vi "INTELLIFAUCET Driver.vi"(0 "Test Fixture Hardware":T2={"Power "={"Yokogawa"={"WT210"={"Sample Rate (1: 0.25s)"=1, "A Range (12: 20A)"=11, "V Range (6: 600V)"=4, "Power VISA Yokogawa WT210"="WT210"}, "WT500"={"Power VISA Yokogawa WT500"="", "V Range (8: 1000V)"=6, "I Range (7: 40A)"=7, "Update Rate (3: 500ms)"=2}, "WT310_2"={"Sample Rate (1: 0.25s)"=1, "A Range (12: 20A)"=11, "V Range (6: 600V)"=4, "Power VISA Yokogawa WT310_2"="WT310_2"}, "WT310_3"={"Sample Rate (1: 0.25s)"=1, "A Range (12: 20A)"=11, "V Range (6: 600V)"=4, "Power VISA Yokogawa WT310_3"="WT310_3"}}, "Aplus"={"Aplus IP Address"="192.168.1.101", "Remote Port"=502, "Instrument"="APLUS", "Instr Driver Revision"="1.03.0053"}, "Power Limits"={"Crest Factor"={"Upper Limit"=1.49, "Lower Limit"=1.34}, "Harmonic Content"={"Uthd"=2.0}, "Voltage"={"% Error"=2.0}, "Stability"={"<1 Watt "={"Wattage"=1.0, "Slope (mW/H)"=10.0}, ">1 Watt"={"1%Power/Hour"=1.0}}}, "Nominal Voltage"=120, "Time Limit (s)"=10800.0, "Power Variation Limit (%)"=50.0, "Power Supply"={"Chroma 61605"="CHROMA", "Use Chroma?"=FALSE}}, "Weight Scale"={"Com Options"={"IND560Scale VISA"="IND560", "IP Address"="", "Remote Port"=502, "Setra Scale VISA"="SETRA", "GSE 350"="GSE350"}, "Select Scale"=""}, "Flow Rates"={"Laurel Cold IP Address"="", "Laurel Hot IP Address"="", "Hot Water Laurel VISA"="LaurelMeter_Hot", "Cold Water Laurel VISA"="LaurelMeter_Cold", "Remote Port"=0, "Laurel Communication Type"="", "Meters To Collect (Hot Cold)"="", "HOT Laurel Reference"=refnum, "COLD Laurel Reference"=refnum}, "Analog Data"={"Agilent"={"Agilent 34972_1"="34972A_1", "Agilent 34972_2"="34972A_2", "Agilent 34972_3"="34972A_3", "Agilent 34972_4"="34972A_3", "Agilent 34972_5"="34972A_3", "Agilent 34972_6"="34972A_3", "Agilent Gain"=0.0, "TC Type (K,J,T)"="", "Instrument IDN?"="", "TC Channels-List"="", "Analog Channels-List"="", "Agilent Cluster Array"=[], "TC Channels-List 2"="", "Analog Channels-List 2"=""}, "Yokogawa"={"MW100"="MW100", "Intellifaucet"=FALSE}, "Select Analog"="", "TC Coefficients"={"TC Coefficients 1"=[], "TC Coefficients 2"=[], "TC Coefficients 3"=[], "TC Coefficients 4"=[], "TC Coefficients 5"=[], "TC Coefficients 6"=[], "TC Coefficients 7"=[]}, "NI Tasks (Dryer DOE)"=["TC Temps-Module 1", "TC Temps-Module 2", "TC Temps-Module 3", "TC Temps-Module 4", "TC Temps-Module 5", "Gas and Temp-Module 6", "AC_DC Events-Module 7"], "Laurel Analog"={"Laurel IP (Water Temp)"="", "Laurel IP (Pressure)"=""}}, "ITHX-Temp Humidity"={"IP Address 1"="", "Remote Port"=0, "IP Address 2"="", "IP Address 3"=""}, "Gas Meter"={"Gas Meter 1"="GasMeter1", "Gas Meter 2"="COM4", "Gas Meter 3"="COM5", "Gas Meter 4"="COM6", "Gas Meter 5"="COM7", "Gas Meter 6"="COM8", "Data Frame Format"={"Absolute Pressure"=FALSE, "Gauge/Diff. Pressure"=FALSE, "Barometric Pressure"=FALSE, "Temperature"=FALSE, "Volumetric"=FALSE, "Mass"=FALSE, "Setpoint"=FALSE, "Valve Drive"=FALSE, "Totalizer"=FALSE, "Totalizer Timer"=FALSE, "Totalizer Average Flow"=FALSE, "Totalizer Peak Flow"=FALSE, "Gas Selected"=FALSE, "Tot. Timer Format"=0}, "Measurement Data"={"Absolute Pressure"=0.0, "Gauge/Diff. Pressure"=0.0, "Barometric Pressure"=0.0, "Temperature"=0.0, "Volumetric Flow"=0.0, "Mass Flow"=0.0, "Setpoint"=0.0, "Valve Drive"=0.0, "Totalizer"=0.0, "[hr]"=0.0, "[min]"=0.0, "[sec]"=0.0, "Totalizer Average Flow"=0.0, "Totalizer Peak Flow"=0.0, "Gas selected"=""}, "Measurement Units"={"Software Rev"="", "Model Number"="", "Manufacturer Info"="", "Software Sub-Rev"="", "Board Rev"="", "Units of Measure Input"={"Abs. Pressure"="", "Gauge/Diff. Press."="", "Barometric Press."="", "Temperature"="", "Volume"="", "Mass"="", "Setpoint"="", "Valve Drive"="", "Totalizer"="", "Tot. Timer"="", "Tot. Avg. Flow"="", "Tot. Peak Flow"=""}}}, "Barometric Pressure"={"HEISE 901A"="HEISE", "Use Barometer?"=FALSE}, "Gas Analysis"={"Ultramat 23 VISA"="ULTRAMAT"}, "Inficon Micro GC"={"Propane IP Address"="192.168.1.33", "Natural Gas  IP Address"="192.168.1.32", "Remote Port"=502}} {"Power"."Yokogawa"."WT310_3"."V Range (6: 600V)" items=["Auto", "15V", "30V", "60V", "150V", "300V", "600V"]; "Power"."Yokogawa"."WT310_3"."A Range (12: 20A)" items=["Auto", "5mA", "10mA", "20mA", "50mA", "100mA", "200mA", "0.5A", "1A", "2A", "5A", "10A", "20A", "50mV", "100mV", "200mV", "2.5V", "5V", "10V"]; "Power"."Yokogawa"."WT310_3"."Sample Rate (1: 0.25s)" items=["0.1s", "0.25s", "0.5s", "1s", "2s", "5s"]; "Power"."Yokogawa"."WT310_2"."V Range (6: 600V)" items=["Auto", "15V", "30V", "60V", "150V", "300V", "600V"]; "Power"."Yokogawa"."WT310_2"."A Range (12: 20A)" items=["Auto", "5mA", "10mA", "20mA", "50mA", "100mA", "200mA", "0.5A", "1A", "2A", "5A", "10A", "20A", "50mV", "100mV", "200mV", "2.5V", "5V", "10V"]; "Power"."Yokogawa"."WT310_2"."Sample Rate (1: 0.25s)" items=["0.1s", "0.25s", "0.5s", "1s", "2s", "5s"]; "Power"."Yokogawa"."WT500"."Update Rate (3: 500ms)" items=["-", "100ms", "200ms", "500ms", "1s", "2s", "5s"]; "Power"."Yokogawa"."WT500"."I Range (7: 40A)" items=["AUTO", "500 mA", "1 A", "2 A", "5 A", "10 A", "20 A", "40 A", "S-AUTO", "50 mV", "100 mV", "200 mV", "500 mV", "1 V", "2 V", "5 V", "10 V", "250 mA", "500 mA", "1 A", "2.5 A", "5 A", "10 A", "20 A", "25 mV", "50 mV", "100 mV", "250 mV", "500 mV", "1 V", "2.5 V", "5 V"]; "Power"."Yokogawa"."WT500"."V Range (8: 1000V)" items=["AUTO", "15", "30", "60", "100", "150", "300", "600", "1000", "7.5", "15", "30", "50", "75", "150", "300", "500"]; "Power"."Yokogawa"."WT210"."V Range (6: 600V)" items=["Auto", "15V", "30V", "60V", "150V", "300V", "600V"]; "Power"."Yokogawa"."WT210"."A Range (12: 20A)" items=["Auto", "5mA", "10mA", "20mA", "50mA", "100mA", "200mA", "0.5A", "1A", "2A", "5A", "10A", "20A", "50mV", "100mV", "200mV", "2.5V", "5V", "10V"]; "Power"."Yokogawa"."WT210"."Sample Rate (1: 0.25s)" items=["0.1s", "0.25s", "0.5s", "1s", "2s", "5s"]}, 1 "Mode":T13=enum."Stop Flow", 2 "Use General Conversion":bool, 3 "TEMP,FLOW":T1, 5 "Temperature(F)":dbl(slide)=58.0 scale=40.0..120.0, 7 "Flow Rate (GPM)":dbl(slide)=100.0 scale=0.0..100.0, 9 "uA Set":i32, 11 "Error In":errorcluster, 12 "Debug":bool, 13 "Refnum in":T12, 14 "Use Proportion Valve":bool) -> (4 "Test Fixture Hardware Output":T2={"Power "={"Yokogawa"={"WT210"={"Sample Rate (1: 0.25s)"=1, "A Range (12: 20A)"=11, "V Range (6: 600V)"=4, "Power VISA Yokogawa WT210"="WT210"}, "WT500"={"Power VISA Yokogawa WT500"="", "V Range (8: 1000V)"=6, "I Range (7: 40A)"=7, "Update Rate (3: 500ms)"=2}, "WT310_2"={"Sample Rate (1: 0.25s)"=1, "A Range (12: 20A)"=11, "V Range (6: 600V)"=4, "Power VISA Yokogawa WT310_2"="WT310_2"}, "WT310_3"={"Sample Rate (1: 0.25s)"=1, "A Range (12: 20A)"=11, "V Range (6: 600V)"=4, "Power VISA Yokogawa WT310_3"="WT310_3"}}, "Aplus"={"Aplus IP Address"="192.168.1.101", "Remote Port"=502, "Instrument"="APLUS", "Instr Driver Revision"="1.03.0053"}, "Power Limits"={"Crest Factor"={"Upper Limit"=1.49, "Lower Limit"=1.34}, "Harmonic Content"={"Uthd"=2.0}, "Voltage"={"% Error"=2.0}, "Stability"={"<1 Watt "={"Wattage"=1.0, "Slope (mW/H)"=10.0}, ">1 Watt"={"1%Power/Hour"=1.0}}}, "Nominal Voltage"=120, "Time Limit (s)"=10800.0, "Power Variation Limit (%)"=50.0, "Power Supply"={"Chroma 61605"="CHROMA", "Use Chroma?"=FALSE}}, "Weight Scale"={"Com Options"={"IND560Scale VISA"="IND560", "IP Address"="", "Remote Port"=502, "Setra Scale VISA"="SETRA", "GSE 350"="GSE350"}, "Select Scale"=""}, "Flow Rates"={"Laurel Cold IP Address"="", "Laurel Hot IP Address"="", "Hot Water Laurel VISA"="LaurelMeter_Hot", "Cold Water Laurel VISA"="LaurelMeter_Cold", "Remote Port"=0, "Laurel Communication Type"="", "Meters To Collect (Hot Cold)"="", "HOT Laurel Reference"=refnum, "COLD Laurel Reference"=refnum}, "Analog Data"={"Agilent"={"Agilent 34972_1"="34972A_1", "Agilent 34972_2"="34972A_2", "Agilent 34972_3"="34972A_3", "Agilent 34972_4"="34972A_3", "Agilent 34972_5"="34972A_3", "Agilent 34972_6"="34972A_3", "Agilent Gain"=0.0, "TC Type (K,J,T)"="", "Instrument IDN?"="", "TC Channels-List"="", "Analog Channels-List"="", "Agilent Cluster Array"=[], "TC Channels-List 2"="", "Analog Channels-List 2"=""}, "Yokogawa"={"MW100"="MW100", "Intellifaucet"=FALSE}, "Select Analog"="", "TC Coefficients"={"TC Coefficients 1"=[], "TC Coefficients 2"=[], "TC Coefficients 3"=[], "TC Coefficients 4"=[], "TC Coefficients 5"=[], "TC Coefficients 6"=[], "TC Coefficients 7"=[]}, "NI Tasks (Dryer DOE)"=["TC Temps-Module 1", "TC Temps-Module 2", "TC Temps-Module 3", "TC Temps-Module 4", "TC Temps-Module 5", "Gas and Temp-Module 6", "AC_DC Events-Module 7"], "Laurel Analog"={"Laurel IP (Water Temp)"="", "Laurel IP (Pressure)"=""}}, "ITHX-Temp Humidity"={"IP Address 1"="", "Remote Port"=0, "IP Address 2"="", "IP Address 3"=""}, "Gas Meter"={"Gas Meter 1"="GasMeter1", "Gas Meter 2"="COM4", "Gas Meter 3"="COM5", "Gas Meter 4"="COM6", "Gas Meter 5"="COM7", "Gas Meter 6"="COM8", "Data Frame Format"={"Absolute Pressure"=FALSE, "Gauge/Diff. Pressure"=FALSE, "Barometric Pressure"=FALSE, "Temperature"=FALSE, "Volumetric"=FALSE, "Mass"=FALSE, "Setpoint"=FALSE, "Valve Drive"=FALSE, "Totalizer"=FALSE, "Totalizer Timer"=FALSE, "Totalizer Average Flow"=FALSE, "Totalizer Peak Flow"=FALSE, "Gas Selected"=FALSE, "Tot. Timer Format"=0}, "Measurement Data"={"Absolute Pressure"=0.0, "Gauge/Diff. Pressure"=0.0, "Barometric Pressure"=0.0, "Temperature"=0.0, "Volumetric Flow"=0.0, "Mass Flow"=0.0, "Setpoint"=0.0, "Valve Drive"=0.0, "Totalizer"=0.0, "[hr]"=0.0, "[min]"=0.0, "[sec]"=0.0, "Totalizer Average Flow"=0.0, "Totalizer Peak Flow"=0.0, "Gas selected"=""}, "Measurement Units"={"Software Rev"="", "Model Number"="", "Manufacturer Info"="", "Software Sub-Rev"="", "Board Rev"="", "Units of Measure Input"={"Abs. Pressure"="", "Gauge/Diff. Press."="", "Barometric Press."="", "Temperature"="", "Volume"="", "Mass"="", "Setpoint"="", "Valve Drive"="", "Totalizer"="", "Tot. Timer"="", "Tot. Avg. Flow"="", "Tot. Peak Flow"=""}}}, "Barometric Pressure"={"HEISE 901A"="HEISE", "Use Barometer?"=FALSE}, "Gas Analysis"={"Ultramat 23 VISA"="ULTRAMAT"}, "Inficon Micro GC"={"Propane IP Address"="192.168.1.33", "Natural Gas  IP Address"="192.168.1.32", "Remote Port"=502}} {"Power"."Yokogawa"."WT310_3"."V Range (6: 600V)" items=["Auto", "15V", "30V", "60V", "150V", "300V", "600V"]; "Power"."Yokogawa"."WT310_3"."A Range (12: 20A)" items=["Auto", "5mA", "10mA", "20mA", "50mA", "100mA", "200mA", "0.5A", "1A", "2A", "5A", "10A", "20A", "50mV", "100mV", "200mV", "2.5V", "5V", "10V"]; "Power"."Yokogawa"."WT310_3"."Sample Rate (1: 0.25s)" items=["0.1s", "0.25s", "0.5s", "1s", "2s", "5s"]; "Power"."Yokogawa"."WT310_2"."V Range (6: 600V)" items=["Auto", "15V", "30V", "60V", "150V", "300V", "600V"]; "Power"."Yokogawa"."WT310_2"."A Range (12: 20A)" items=["Auto", "5mA", "10mA", "20mA", "50mA", "100mA", "200mA", "0.5A", "1A", "2A", "5A", "10A", "20A", "50mV", "100mV", "200mV", "2.5V", "5V", "10V"]; "Power"."Yokogawa"."WT310_2"."Sample Rate (1: 0.25s)" items=["0.1s", "0.25s", "0.5s", "1s", "2s", "5s"]; "Power"."Yokogawa"."WT500"."Update Rate (3: 500ms)" items=["-", "100ms", "200ms", "500ms", "1s", "2s", "5s"]; "Power"."Yokogawa"."WT500"."I Range (7: 40A)" items=["AUTO", "500 mA", "1 A", "2 A", "5 A", "10 A", "20 A", "40 A", "S-AUTO", "50 mV", "100 mV", "200 mV", "500 mV", "1 V", "2 V", "5 V", "10 V", "250 mA", "500 mA", "1 A", "2.5 A", "5 A", "10 A", "20 A", "25 mV", "50 mV", "100 mV", "250 mV", "500 mV", "1 V", "2.5 V", "5 V"]; "Power"."Yokogawa"."WT500"."V Range (8: 1000V)" items=["AUTO", "15", "30", "60", "100", "150", "300", "600", "1000", "7.5", "15", "30", "50", "75", "150", "300", "500"]; "Power"."Yokogawa"."WT210"."V Range (6: 600V)" items=["Auto", "15V", "30V", "60V", "150V", "300V", "600V"]; "Power"."Yokogawa"."WT210"."A Range (12: 20A)" items=["Auto", "5mA", "10mA", "20mA", "50mA", "100mA", "200mA", "0.5A", "1A", "2A", "5A", "10A", "20A", "50mV", "100mV", "200mV", "2.5V", "5V", "10V"]; "Power"."Yokogawa"."WT210"."Sample Rate (1: 0.25s)" items=["0.1s", "0.25s", "0.5s", "1s", "2s", "5s"]}, 8 "uA Output":i32, 15 "Error Out":errorcluster)   [LabVIEW 2019]
uses:
  Type Definitions/INTELLIFAUCET Set Mode.ctl
  Washer DOE/Type Definitions/DOE Test Fixture Hardware.ctl
  Utility/Type Definitions/UTILITY Power Inputs Control.ctl
  Drivers/IND560 Scale Monitor/Type Definitions/IND560 Configuration.ctl
  Type Definitions/HEWH Agilent Cluster.ctl
  Utility/Type Definitions/UTILITY TC Coefficients.ctl
  Drivers/Omega FMA-1600A Series Gas Flow Meter/Type Definitions/FMA1600A COM Ports.ctl
  Drivers/Alicat Gas Meter Driver/Sub-VIs/Data Frame.ctl
  Drivers/Alicat Gas Meter Driver/Sub-VIs/Data Cluster.ctl
  Drivers/Omega FMA-1600A Series Gas Flow Meter/Type Definitions/FMA1600A Units String.ctl
  Drivers/Alicat Gas Meter Driver/Sub-VIs/Units of Measure.ctl
  Type Definitions/INTELLIFAUCT Temp Flow.ctl
panel:
  in  "milliseconds to wait":u32=75
  # "%"
  # "Totalizer Timer"
  # "Totalizer Timer"
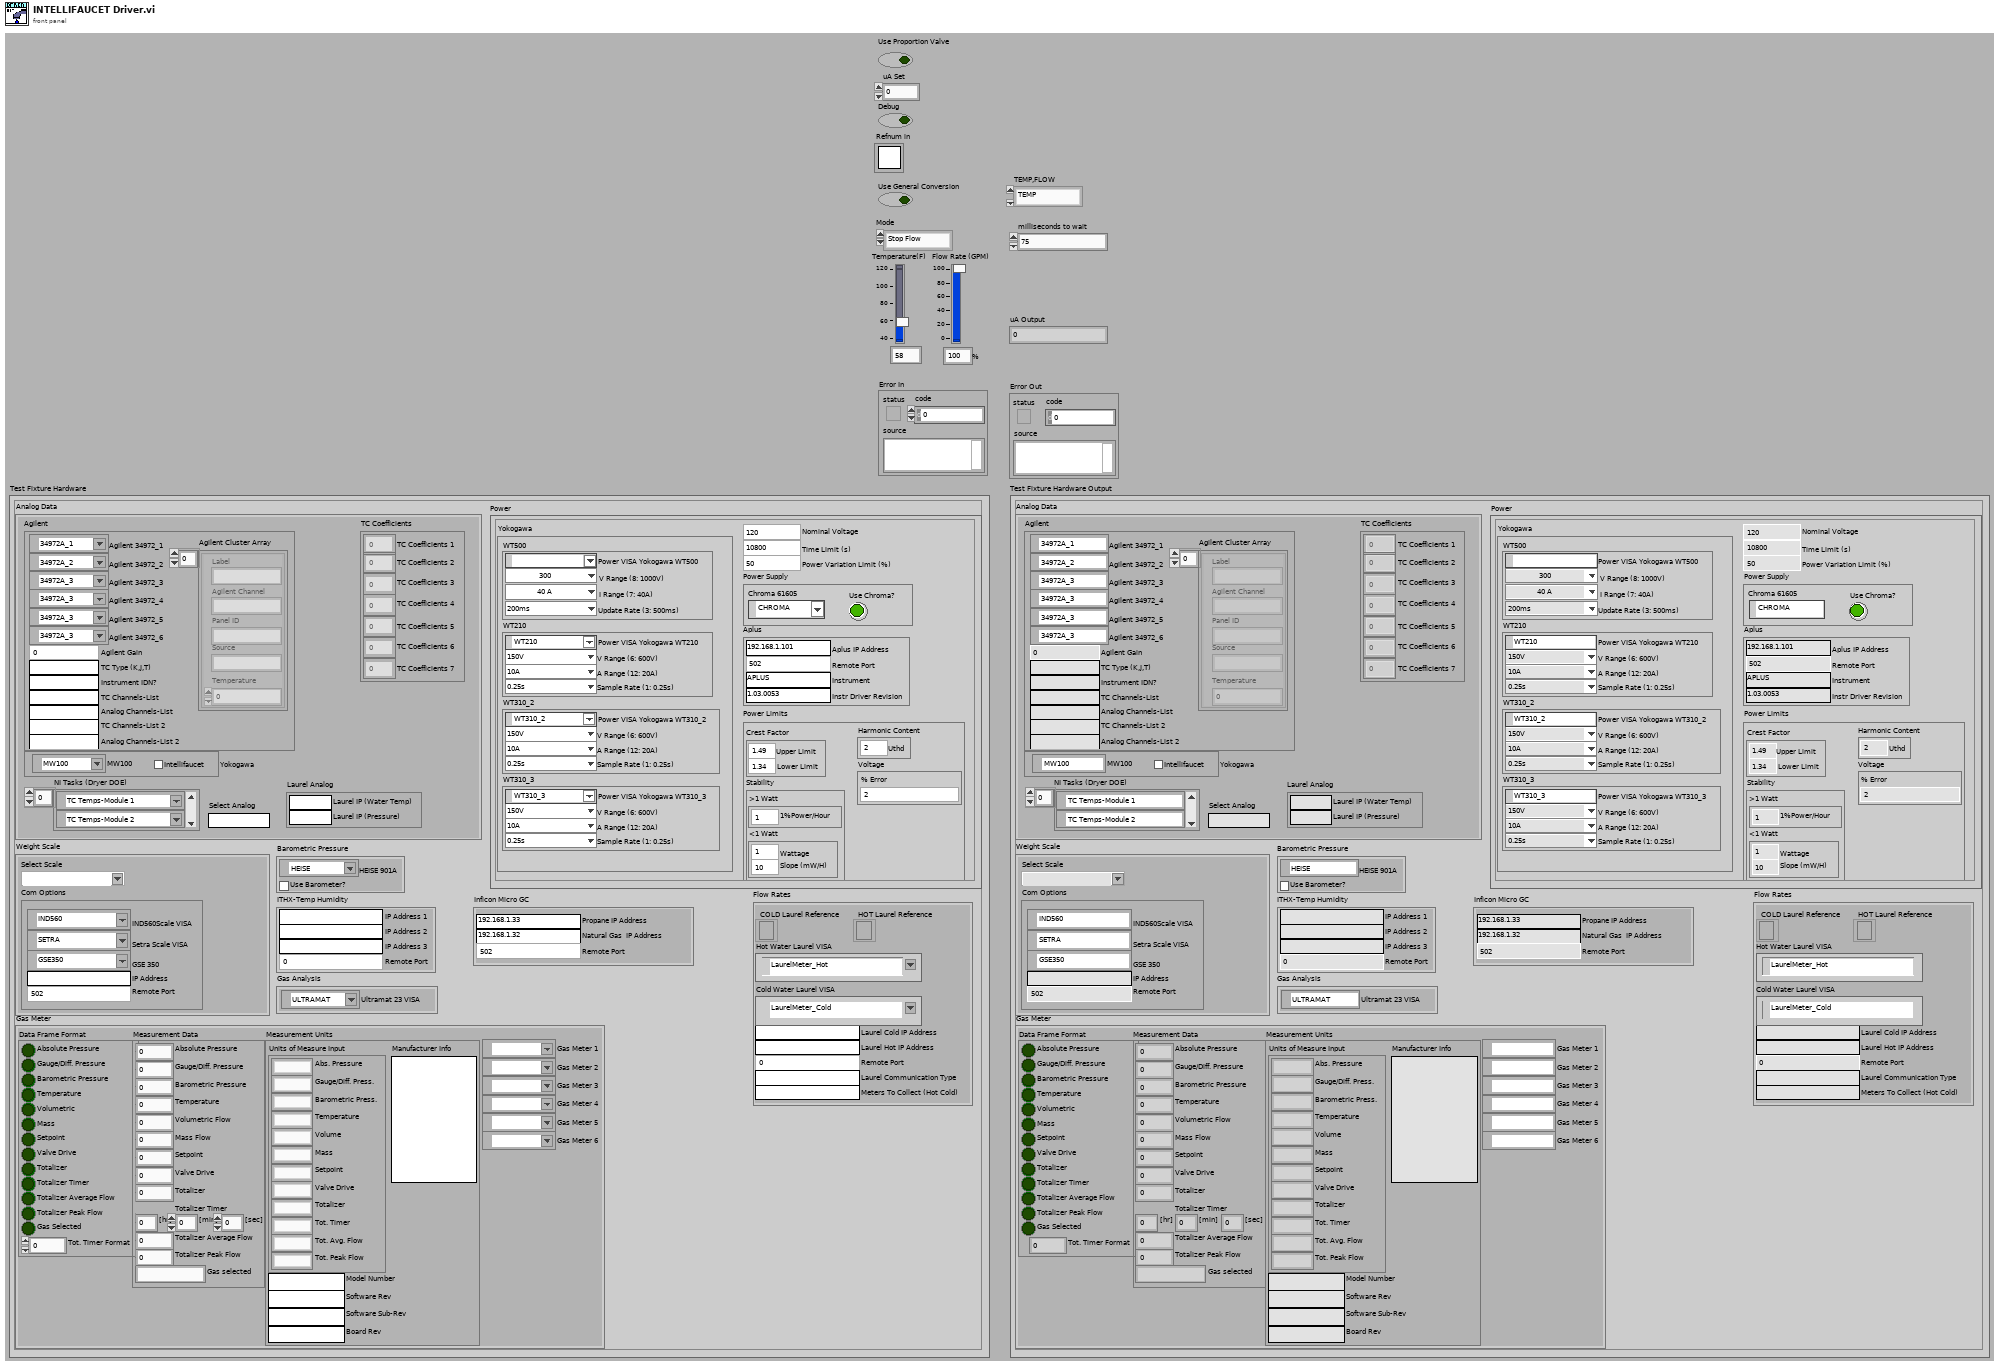
[diagram p1: front panel]
types:
  T1 = typedef "INTELLIFAUCT Temp Flow.ctl" = enum8{"TEMP", "FLOW"}
  T2 = typedef "DOE Test Fixture Hardware.ctl" = cluster{"Power ":T3, "Weight Scale":cluster{"Com Options":T4, "Select Scale":string}, "Flow Rates":cluster{"Laurel Cold IP Address":string, "Laurel Hot IP Address":string, "Hot Water Laurel VISA":refnum<visa-resource-name>, "Cold Water Laurel VISA":refnum<visa-resource-name>, "Remote Port":u16, "Laurel Communication Type":string, "Meters To Collect (Hot Cold)":string, "HOT Laurel Reference":refnum<k5>, "COLD Laurel Reference":refnum<k5>}, "Analog Data":cluster{"Agilent":cluster{"Agilent 34972_1":refnum<visa-resource-name>, "Agilent 34972_2":refnum<visa-resource-name>, "Agilent 34972_3":refnum<visa-resource-name>, "Agilent 34972_4":refnum<visa-resource-name>, "Agilent 34972_5":refnum<visa-resource-name>, "Agilent 34972_6":refnum<visa-resource-name>, "Agilent Gain":dbl, "TC Type (K,J,T)":string, "Instrument IDN?":string, "TC Channels-List":string, "Analog Channels-List":string, "Agilent Cluster Array":T5[], "TC Channels-List 2":string, "Analog Channels-List 2":string}, "Yokogawa":cluster{"MW100":refnum<visa-resource-name>, "Intellifaucet":bool}, "Select Analog":string, "TC Coefficients":T6, "NI Tasks (Dryer DOE)":refnum<k21>[], "Laurel Analog":cluster{"Laurel IP (Water Temp)":string, "Laurel IP (Pressure)":string}}, "ITHX-Temp Humidity":cluster{"IP Address 1":string, "Remote Port":u16, "IP Address 2":string, "IP Address 3":string}, "Gas Meter":T7, "Barometric Pressure":cluster{"HEISE 901A":refnum<visa-resource-name>, "Use Barometer?":bool}, "Gas Analysis":cluster{"Ultramat 23 VISA":refnum<visa-resource-name>}, "Inficon Micro GC":cluster{"Propane IP Address":string, "Natural Gas  IP Address":string, "Remote Port":u16}}
  T3 = typedef "UTILITY Power Inputs Control.ctl" = cluster{"Yokogawa":cluster{"WT210":cluster{"Sample Rate (1: 0.25s)":i32, "A Range (12: 20A)":i32, "V Range (6: 600V)":i32, "Power VISA Yokogawa WT210":refnum<visa-resource-name>}, "WT500":cluster{"Power VISA Yokogawa WT500":refnum<visa-resource-name>, "V Range (8: 1000V)":i32, "I Range (7: 40A)":i32, "Update Rate (3: 500ms)":i32}, "WT310_2":cluster{"Sample Rate (1: 0.25s)":i32, "A Range (12: 20A)":i32, "V Range (6: 600V)":i32, "Power VISA Yokogawa WT310_2":refnum<visa-resource-name>}, "WT310_3":cluster{"Sample Rate (1: 0.25s)":i32, "A Range (12: 20A)":i32, "V Range (6: 600V)":i32, "Power VISA Yokogawa WT310_3":refnum<visa-resource-name>}}, "Aplus":cluster{"Aplus IP Address":string, "Remote Port":i32, "Instrument":string, "Instr Driver Revision":string}, "Power Limits":cluster{"Crest Factor":cluster{"Upper Limit":dbl, "Lower Limit":dbl}, "Harmonic Content":cluster{"Uthd":dbl}, "Voltage":cluster{"% Error":dbl}, "Stability":cluster{"<1 Watt ":cluster{"Wattage":dbl, "Slope (mW/H)":dbl}, ">1 Watt":cluster{"1%Power/Hour":dbl}}}, "Nominal Voltage":i32, "Time Limit (s)":dbl, "Power Variation Limit (%)":dbl, "Power Supply":cluster{"Chroma 61605":refnum<visa-resource-name>, "Use Chroma?":bool}}
  T4 = typedef "IND560 Configuration.ctl" = cluster{"IND560Scale VISA":refnum<visa-resource-name>, "IP Address":string, "Remote Port":u16, "Setra Scale VISA":refnum<visa-resource-name>, "GSE 350":refnum<visa-resource-name>}
  T5 = typedef "HEWH Agilent Cluster.ctl" = cluster{"Label":string, "Agilent Channel":string, "Panel ID":string, "Source":string, "Temperature":dbl}
  T6 = typedef "UTILITY TC Coefficients.ctl" = cluster{"TC Coefficients 1":dbl[], "TC Coefficients 2":dbl[], "TC Coefficients 3":dbl[], "TC Coefficients 4":dbl[], "TC Coefficients 5":dbl[], "TC Coefficients 6":dbl[], "TC Coefficients 7":dbl[]}
  T7 = typedef "FMA1600A COM Ports.ctl" = cluster{"Gas Meter 1":refnum<visa-resource-name>, "Gas Meter 2":refnum<visa-resource-name>, "Gas Meter 3":refnum<visa-resource-name>, "Gas Meter 4":refnum<visa-resource-name>, "Gas Meter 5":refnum<visa-resource-name>, "Gas Meter 6":refnum<visa-resource-name>, "Data Frame Format":T8, "Measurement Data":T9, "Measurement Units":T10}
  T8 = typedef "Data Frame.ctl" = cluster{"Absolute Pressure":bool, "Gauge/Diff. Pressure":bool, "Barometric Pressure":bool, "Temperature":bool, "Volumetric":bool, "Mass":bool, "Setpoint":bool, "Valve Drive":bool, "Totalizer":bool, "Totalizer Timer":bool, "Totalizer Average Flow":bool, "Totalizer Peak Flow":bool, "Gas Selected":bool, "Tot. Timer Format":u16}
  T9 = typedef "Data Cluster.ctl" = cluster{"Absolute Pressure":dbl, "Gauge/Diff. Pressure":dbl, "Barometric Pressure":dbl, "Temperature":dbl, "Volumetric Flow":dbl, "Mass Flow":dbl, "Setpoint":dbl, "Valve Drive":dbl, "Totalizer":dbl, "[hr]":dbl, "[min]":dbl, "[sec]":dbl, "Totalizer Average Flow":dbl, "Totalizer Peak Flow":dbl, "Gas selected":string}
  T10 = typedef "FMA1600A Units String.ctl" = cluster{"Software Rev":string, "Model Number":string, "Manufacturer Info":string, "Software Sub-Rev":string, "Board Rev":string, "Units of Measure Input":T11}
  T11 = typedef "Units of Measure.ctl" = cluster{"Abs. Pressure":string, "Gauge/Diff. Press.":string, "Barometric Press.":string, "Temperature":string, "Volume":string, "Mass":string, "Setpoint":string, "Valve Drive":string, "Totalizer":string, "Tot. Timer":string, "Tot. Avg. Flow":string, "Tot. Peak Flow":string}
  T12 = typedef "Semaphore RefNum" = refnum<k1>
  T13 = typedef "INTELLIFAUCET Set Mode.ctl" = enum16{"Adjust Temp", "Adjust Flow", "Start Flow", "Stop Flow", "Hold Start", "Hold Stop", "Release Start", "Release Stop", "Temp/Flow Relay"}
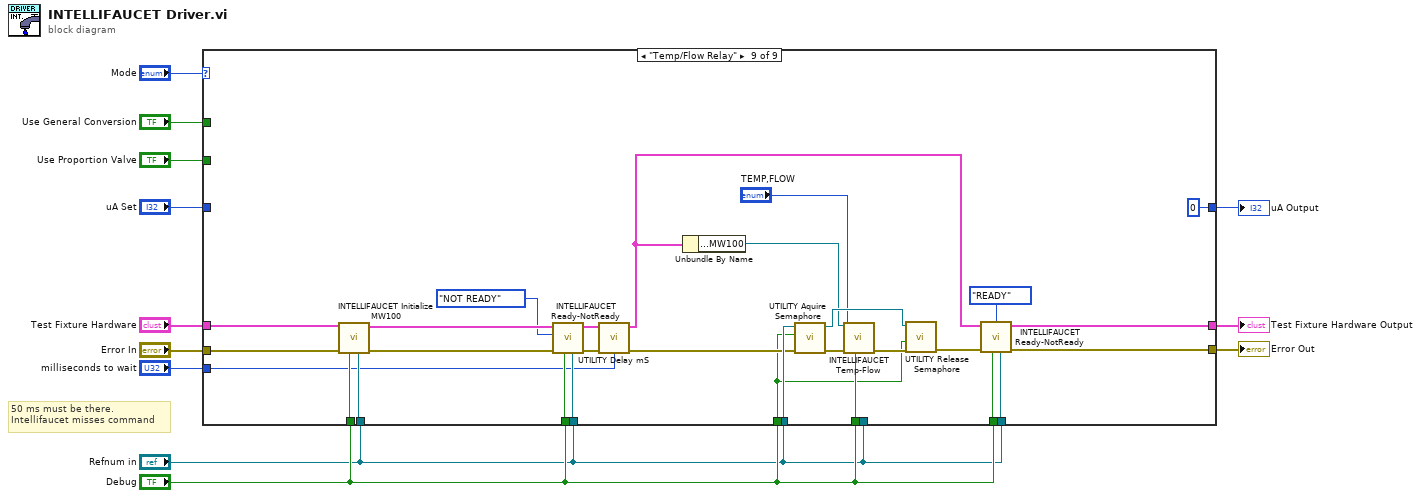
[diagram p0: block diagram]
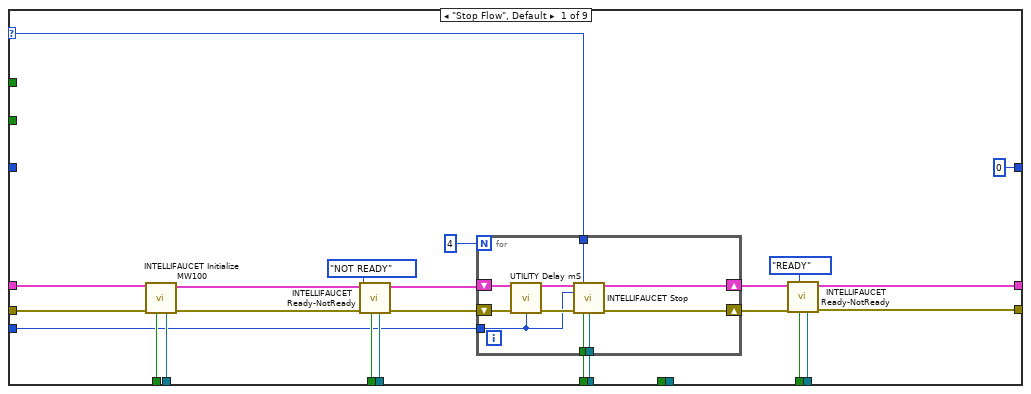
[diagram p2: hidden frame]
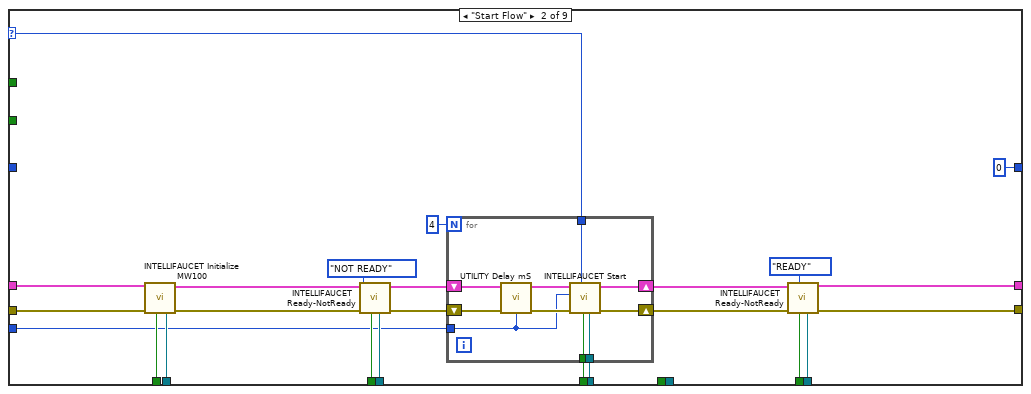
[diagram p3: hidden frame]
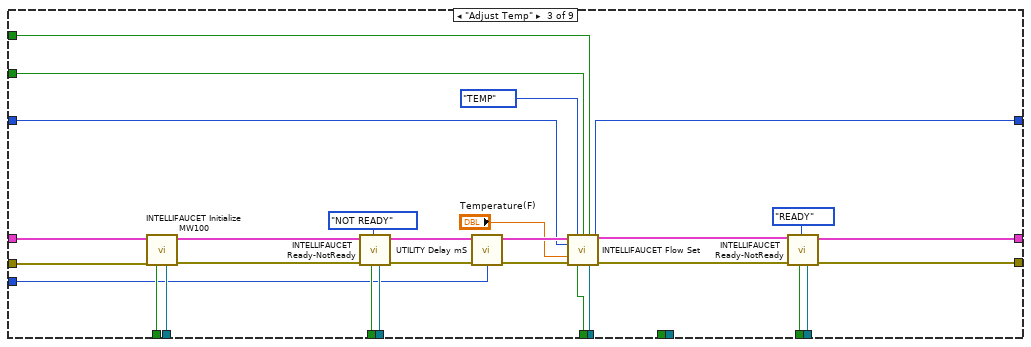
[diagram p4: hidden frame]
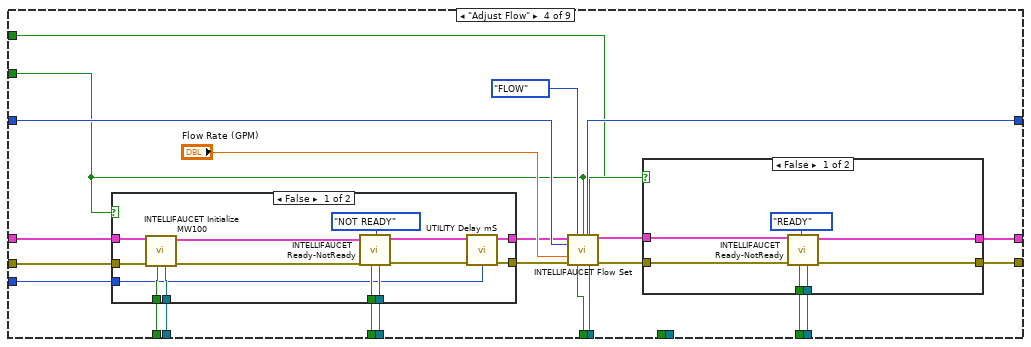
[diagram p5: hidden frame]
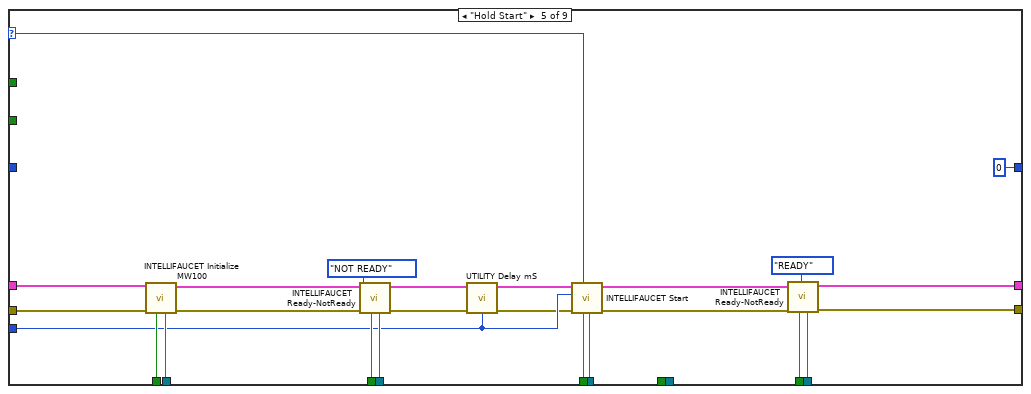
[diagram p8: hidden frame]
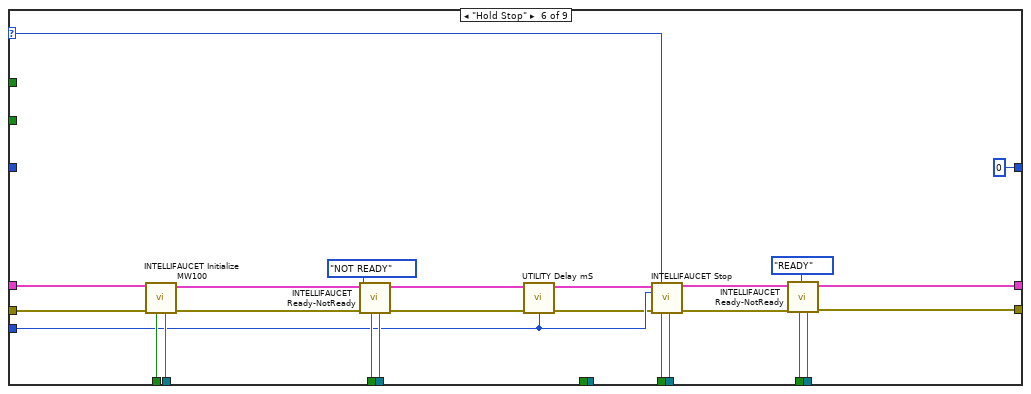
[diagram p9: hidden frame]
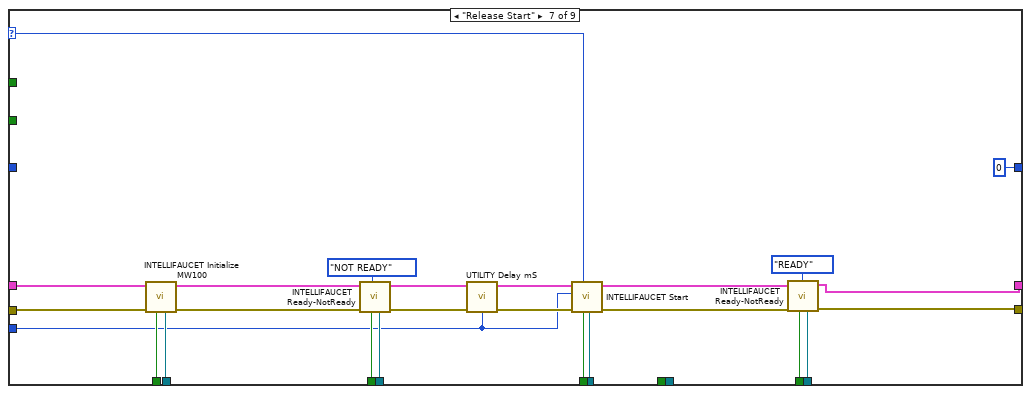
[diagram p10: hidden frame]
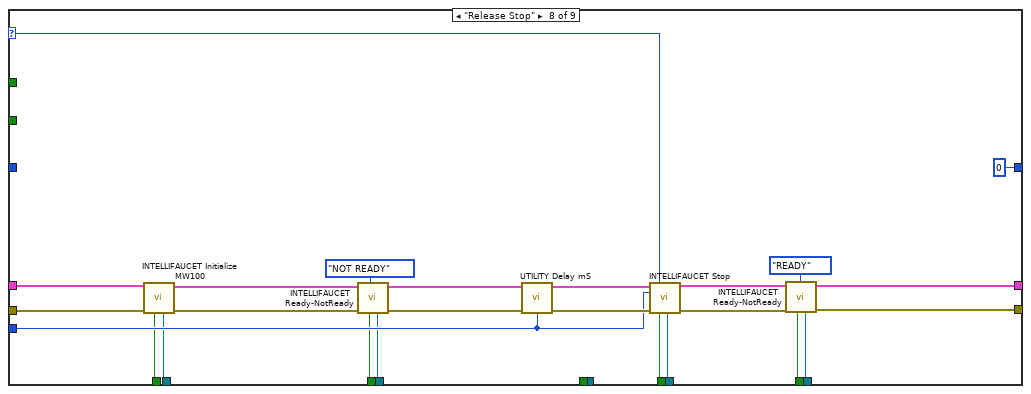
[diagram p11: hidden frame]
diagram:
  # "50 ms must be there.\nIntellifaucet misses command"
  n1 = case shown="\"Temp/Flow Relay\"" "Mode" {
    selector: "Mode" -> [w13 w46 _ _ w154 w178 w203 w226 _]
    tunnel: "milliseconds to wait" -> [w15 w48 w86 w115 w161 w185 w204 w240 w263]
    tunnel: [w19 w57 w82 w127 w165 w189 w213 w236 w272] -> w10
    tunnel: "Test Fixture Hardware" -> [w35 w69 w101 w129 w172 w196 w215 w239 w271]
    tunnel: "Error In" -> [w36 w68 w102 w124 w171 w195 w216 w238 w270]
    tunnel: [w20 w56 w99 w128 w166 w190 w214 w237 w273] -> w2
    tunnel: "Debug" -> [w28 w55 w96 w122 w168 w192 w207 w231 w267]
    tunnel: "Refnum in" -> [w27 w54 w95 w123 w167 w191 w208 w230 w266]
    tunnel: "Refnum in" -> [w33 w67 w97 w126 w169 w193 w206 w229 w268]
    tunnel: "Debug" -> [w34 w66 w98 w125 w170 w194 w205 w228 w269]
    tunnel: "Refnum in" -> [w31 w64 w93 w121 w157 _ w210 _ w260]
    tunnel: "Debug" -> [w32 w65 w94 w120 w158 _ w209 _ w254]
    tunnel: "Debug" -> [w18 w53 w92 w119 w164 w188 w212 w235 w265]
    tunnel: "Refnum in" -> [w17 w52 w91 w118 w163 w187 w211 w234 w264]
    tunnel: [0 ("uA Output") 0 ("uA Output") w90 w117 0 ("uA Output") 0 ("uA Output") 0 ("uA Output") 0 ("uA Output") 0 ("uA Output")] -> w9
    tunnel: "uA Set" -> [_ _ w89 w116 _ _ _ _ _]
    tunnel: "Use Proportion Valve" -> [_ _ w83 w108 _ _ _ _ _]
    tunnel: "Debug" -> [_ _ _ _ _ w182 _ w233 w262]
    tunnel: "Refnum in" -> [_ _ _ _ _ w181 _ w232 _]
    tunnel: "Use General Conversion" -> [_ _ w79 w107 _ _ _ _ _]
    frame "Stop Flow", Default {
      n2 = call "INTELLIFAUCET Initialize MW100.vi"("Refnum in"=w33, "Debug"=w34, "error in (no error)"=w36, "Test Fixture Hardware"=w35) -> ("error out"=w26:errorcluster, "Test Fixture Hardware Output"=w24:T2)  [unwired: 6 in]
      n3 = call "INTELLIFAUCET Ready-NotReady.vi"("Refnum in"=w27, "Debug"=w28, "Error In"=w26, "READY?"=enum8{"READY", "NOT READY"}."NOT READY", "Test Fixture Hardware"=w24) -> ("Error Out"=w25:errorcluster, "Test Fixture Hardware Output"=w23:T2)  [unwired: 5 in]
      n4 = for {
        N: 4 -> [_]
        tunnel: w32 -> [w44]
        tunnel: w31 -> [w43]
        tunnel: w15 -> [w39]
        shift-right: [w38] -> w16
        shift-left: w25 -> [w42]
        shift-right: [w40] -> w21
        shift-left: w23 -> [w41]
        tunnel: w13 -> [w37]
        n5 = call "UTILITY Delay mS.vi"("Error In"=w42, "milliseconds to wait"=w39) -> ("Error Out"=w45:errorcluster)  [unwired: 13 in]
        n6 = call "INTELLIFAUCET Stop.vi"("Test Fixture Hardware"=w41, "Mode"=w37, "mS wait"=w39, "Error In"=w45, "Debug"=w44, "Refnum in"=w43) -> ("Test Fixture Hardware Output"=w40:T2, "Error Out"=w38:errorcluster)  [unwired: 8 in]
      }
      n7 = call "INTELLIFAUCET Ready-NotReady.vi"("Refnum in"=w17, "Debug"=w18, "Error In"=w16, "READY?"=enum8{"READY", "NOT READY"}."READY", "Test Fixture Hardware"=w21) -> ("Error Out"=w19:errorcluster, "Test Fixture Hardware Output"=w20:T2)  [unwired: 5 in]
    }
    frame "Start Flow" {
      n8 = call "INTELLIFAUCET Initialize MW100.vi"("Refnum in"=w67, "Debug"=w66, "error in (no error)"=w68, "Test Fixture Hardware"=w69) -> ("error out"=w50:errorcluster, "Test Fixture Hardware Output"=w61:T2)  [unwired: 6 in]
      n9 = call "INTELLIFAUCET Ready-NotReady.vi"("Refnum in"=w54, "Debug"=w55, "Error In"=w50, "READY?"=enum8{"READY", "NOT READY"}."NOT READY", "Test Fixture Hardware"=w61) -> ("Error Out"=w51:errorcluster, "Test Fixture Hardware Output"=w60:T2)  [unwired: 5 in]
      n10 = for {
        N: 4 -> [_]
        tunnel: w65 -> [w78]
        tunnel: w64 -> [w77]
        tunnel: w48 -> [w72]
        shift-right: [w75] -> w58
        shift-left: w60 -> [w76]
        shift-right: [w71] -> w49
        shift-left: w51 -> [w74]
        tunnel: w46 -> [w70]
        n11 = call "UTILITY Delay mS.vi"("Error In"=w74, "milliseconds to wait"=w72) -> ("Error Out"=w73:errorcluster)  [unwired: 13 in]
        n12 = call "INTELLIFAUCET Start.vi"("Refnum in"=w77, "Debug"=w78, "Mode"=w70, "Error In"=w73, "mS wait"=w72, "Test Fixture Hardware"=w76) -> ("Error Out"=w71:errorcluster, "Test Fixture Hardware Output"=w75:T2)  [unwired: 4 in]
      }
      n13 = call "INTELLIFAUCET Ready-NotReady.vi"("Refnum in"=w52, "Debug"=w53, "Error In"=w49, "READY?"=enum8{"READY", "NOT READY"}."READY", "Test Fixture Hardware"=w58) -> ("Error Out"=w57:errorcluster, "Test Fixture Hardware Output"=w56:T2)  [unwired: 5 in]
    }
    frame "Adjust Temp" {
      n14 = call "INTELLIFAUCET Initialize MW100.vi"("Refnum in"=w97, "Debug"=w98, "error in (no error)"=w102, "Test Fixture Hardware"=w101) -> ("error out"=w81:errorcluster, "Test Fixture Hardware Output"=w100:T2)  [unwired: 6 in]
      n15 = call "INTELLIFAUCET Ready-NotReady.vi"("Refnum in"=w95, "Debug"=w96, "Error In"=w81, "READY?"=enum8{"READY", "NOT READY"}."NOT READY", "Test Fixture Hardware"=w100) -> ("Error Out"=w88:errorcluster, "Test Fixture Hardware Output"=w105:T2)  [unwired: 5 in]
      n16 = call "UTILITY Delay mS.vi"("Error In"=w88, "milliseconds to wait"=w86) -> ("Error Out"=w87:errorcluster)  [unwired: 13 in]
      n17 = call "INTELLIFAUCET Flow Set.vi"("Test Fixture Hardware"=w105, "TEMP,FLOW"=INTELLIFAUCT_Temp_Flow."TEMP", "Use Proportion Valve"=w83, "Use General Conversion"=w79, "uA Set"=w89, "Temp/GPM Target"="Temperature(F)", "error in (no error)"=w87, "Debug"=w94, "Refnum in"=w93) -> ("Test Fixture Hardware Output"=w103:T2, "uA Output"=w90:i32, "error out"=w80:errorcluster)  [unwired: 4 in]
      n18 = call "INTELLIFAUCET Ready-NotReady.vi"("Refnum in"=w91, "Debug"=w92, "Error In"=w80, "READY?"=enum8{"READY", "NOT READY"}."READY", "Test Fixture Hardware"=w103) -> ("Error Out"=w82:errorcluster, "Test Fixture Hardware Output"=w99:T2)  [unwired: 5 in]
    }
    frame "Adjust Flow" {
      n19 = case shown="False" w108 {
        tunnel: w129 -> [w151 w152]
        tunnel: w126 -> [w150 _]
        tunnel: w125 -> [w149 _]
        tunnel: w124 -> [w148 w153]
        tunnel: w123 -> [w147 _]
        tunnel: w122 -> [w146 _]
        tunnel: w115 -> [w145 _]
        tunnel: [w143 w152] -> w112
        tunnel: [w141 w153] -> w109
        frame False {
          n20 = call "INTELLIFAUCET Initialize MW100.vi"("Refnum in"=w150, "Debug"=w149, "error in (no error)"=w148, "Test Fixture Hardware"=w151) -> ("error out"=w139:errorcluster, "Test Fixture Hardware Output"=w144:T2)  [unwired: 6 in]
          n21 = call "INTELLIFAUCET Ready-NotReady.vi"("Refnum in"=w147, "Debug"=w146, "Error In"=w139, "READY?"=enum8{"READY", "NOT READY"}."NOT READY", "Test Fixture Hardware"=w144) -> ("Error Out"=w142:errorcluster, "Test Fixture Hardware Output"=w143:T2)  [unwired: 5 in]
          n22 = call "UTILITY Delay mS.vi"("Error In"=w142, "milliseconds to wait"=w145) -> ("Error Out"=w141:errorcluster)  [unwired: 13 in]
        }
        frame True {
        }
      }
      n23 = call "INTELLIFAUCET Flow Set.vi"("Test Fixture Hardware"=w112, "TEMP,FLOW"=INTELLIFAUCT_Temp_Flow."FLOW", "Use Proportion Valve"=w108, "Use General Conversion"=w107, "uA Set"=w116, "Temp/GPM Target"="Flow Rate (GPM)", "error in (no error)"=w109, "Debug"=w120, "Refnum in"=w121) -> ("Test Fixture Hardware Output"=w111:T2, "uA Output"=w117:i32, "error out"=w110:errorcluster)  [unwired: 4 in]
      n24 = case shown="False" w108 {
        tunnel: [w136 w138] -> w128
        tunnel: [w131 w137] -> w127
        tunnel: w119 -> [w135 _]
        tunnel: w118 -> [w134 _]
        tunnel: w111 -> [w133 w138]
        tunnel: w110 -> [w130 w137]
        frame False {
          n25 = call "INTELLIFAUCET Ready-NotReady.vi"("Refnum in"=w134, "Debug"=w135, "Error In"=w130, "READY?"=enum8{"READY", "NOT READY"}."READY", "Test Fixture Hardware"=w133) -> ("Error Out"=w131:errorcluster, "Test Fixture Hardware Output"=w136:T2)  [unwired: 5 in]
        }
        frame True {
        }
      }
    }
    frame "Hold Start" {
      n26 = call "INTELLIFAUCET Initialize MW100.vi"("Refnum in"=w169, "Debug"=w170, "error in (no error)"=w171, "Test Fixture Hardware"=w172) -> ("error out"=w176:errorcluster, "Test Fixture Hardware Output"=w174:T2)  [unwired: 6 in]
      n27 = call "INTELLIFAUCET Ready-NotReady.vi"("Refnum in"=w167, "Debug"=w168, "Error In"=w176, "READY?"=enum8{"READY", "NOT READY"}."NOT READY", "Test Fixture Hardware"=w174) -> ("Error Out"=w175:errorcluster, "Test Fixture Hardware Output"=w159:T2)  [unwired: 5 in]
      n28 = call "UTILITY Delay mS.vi"("Error In"=w175, "milliseconds to wait"=w161) -> ("Error Out"=w160:errorcluster)  [unwired: 13 in]
      n29 = call "INTELLIFAUCET Start.vi"("Refnum in"=w157, "Debug"=w158, "Mode"=w154, "Error In"=w160, "mS wait"=w161, "Test Fixture Hardware"=w159) -> ("Error Out"=w155:errorcluster, "Test Fixture Hardware Output"=w156:T2)  [unwired: 4 in]
      n30 = call "INTELLIFAUCET Ready-NotReady.vi"("Refnum in"=w163, "Debug"=w164, "Error In"=w155, "READY?"=enum8{"READY", "NOT READY"}."READY", "Test Fixture Hardware"=w156) -> ("Error Out"=w165:errorcluster, "Test Fixture Hardware Output"=w166:T2)  [unwired: 5 in]
    }
    frame "Hold Stop" {
      n31 = call "INTELLIFAUCET Initialize MW100.vi"("Refnum in"=w193, "Debug"=w194, "error in (no error)"=w195, "Test Fixture Hardware"=w196) -> ("error out"=w200:errorcluster, "Test Fixture Hardware Output"=w198:T2)  [unwired: 6 in]
      n32 = call "INTELLIFAUCET Ready-NotReady.vi"("Refnum in"=w191, "Debug"=w192, "Error In"=w200, "READY?"=enum8{"READY", "NOT READY"}."NOT READY", "Test Fixture Hardware"=w198) -> ("Error Out"=w199:errorcluster, "Test Fixture Hardware Output"=w179:T2)  [unwired: 5 in]
      n33 = call "UTILITY Delay mS.vi"("Error In"=w199, "milliseconds to wait"=w185) -> ("Error Out"=w180:errorcluster)  [unwired: 13 in]
      n34 = call "INTELLIFAUCET Stop.vi"("Test Fixture Hardware"=w179, "Mode"=w178, "mS wait"=w185, "Error In"=w180, "Debug"=w182, "Refnum in"=w181) -> ("Test Fixture Hardware Output"=w183:T2, "Error Out"=w184:errorcluster)  [unwired: 8 in]
      n35 = call "INTELLIFAUCET Ready-NotReady.vi"("Refnum in"=w187, "Debug"=w188, "Error In"=w184, "READY?"=enum8{"READY", "NOT READY"}."READY", "Test Fixture Hardware"=w183) -> ("Error Out"=w189:errorcluster, "Test Fixture Hardware Output"=w190:T2)  [unwired: 5 in]
    }
    frame "Release Start" {
      n36 = call "INTELLIFAUCET Initialize MW100.vi"("Refnum in"=w206, "Debug"=w205, "error in (no error)"=w216, "Test Fixture Hardware"=w215) -> ("error out"=w225:errorcluster, "Test Fixture Hardware Output"=w223:T2)  [unwired: 6 in]
      n37 = call "INTELLIFAUCET Ready-NotReady.vi"("Refnum in"=w208, "Debug"=w207, "Error In"=w225, "READY?"=enum8{"READY", "NOT READY"}."NOT READY", "Test Fixture Hardware"=w223) -> ("Error Out"=w224:errorcluster, "Test Fixture Hardware Output"=w221:T2)  [unwired: 5 in]
      n38 = call "UTILITY Delay mS.vi"("Error In"=w224, "milliseconds to wait"=w204) -> ("Error Out"=w222:errorcluster)  [unwired: 13 in]
      n39 = call "INTELLIFAUCET Start.vi"("Refnum in"=w210, "Debug"=w209, "Mode"=w203, "Error In"=w222, "mS wait"=w204, "Test Fixture Hardware"=w221) -> ("Error Out"=w219:errorcluster, "Test Fixture Hardware Output"=w220:T2)  [unwired: 4 in]
      n40 = call "INTELLIFAUCET Ready-NotReady.vi"("Refnum in"=w211, "Debug"=w212, "Error In"=w219, "READY?"=enum8{"READY", "NOT READY"}."READY", "Test Fixture Hardware"=w220) -> ("Error Out"=w213:errorcluster, "Test Fixture Hardware Output"=w214:T2)  [unwired: 5 in]
    }
    frame "Release Stop" {
      n41 = call "INTELLIFAUCET Initialize MW100.vi"("Refnum in"=w229, "Debug"=w228, "error in (no error)"=w238, "Test Fixture Hardware"=w239) -> ("error out"=w249:errorcluster, "Test Fixture Hardware Output"=w247:T2)  [unwired: 6 in]
      n42 = call "INTELLIFAUCET Ready-NotReady.vi"("Refnum in"=w230, "Debug"=w231, "Error In"=w249, "READY?"=enum8{"READY", "NOT READY"}."NOT READY", "Test Fixture Hardware"=w247) -> ("Error Out"=w248:errorcluster, "Test Fixture Hardware Output"=w243:T2)  [unwired: 5 in]
      n43 = call "UTILITY Delay mS.vi"("Error In"=w248, "milliseconds to wait"=w240) -> ("Error Out"=w244:errorcluster)  [unwired: 13 in]
      n44 = call "INTELLIFAUCET Stop.vi"("Test Fixture Hardware"=w243, "Mode"=w226, "mS wait"=w240, "Error In"=w244, "Debug"=w233, "Refnum in"=w232) -> ("Test Fixture Hardware Output"=w245:T2, "Error Out"=w246:errorcluster)  [unwired: 8 in]
      n45 = call "INTELLIFAUCET Ready-NotReady.vi"("Refnum in"=w234, "Debug"=w235, "Error In"=w246, "READY?"=enum8{"READY", "NOT READY"}."READY", "Test Fixture Hardware"=w245) -> ("Error Out"=w236:errorcluster, "Test Fixture Hardware Output"=w237:T2)  [unwired: 5 in]
    }
    frame "Temp/Flow Relay" {
      n46 = call "INTELLIFAUCET Initialize MW100.vi"("Refnum in"=w268, "Debug"=w269, "error in (no error)"=w270, "Test Fixture Hardware"=w271) -> ("error out"=w277:errorcluster, "Test Fixture Hardware Output"=w276:T2)  [unwired: 6 in]
      n47 = call "INTELLIFAUCET Ready-NotReady.vi"("Refnum in"=w266, "Debug"=w267, "Error In"=w277, "READY?"=enum8{"READY", "NOT READY"}."NOT READY", "Test Fixture Hardware"=w276) -> ("Error Out"=w261:errorcluster, "Test Fixture Hardware Output"=w251:T2)  [unwired: 5 in]
      n48 = call "UTILITY Delay mS.vi"("Error In"=w261, "milliseconds to wait"=w263) -> ("Error Out"=w258:errorcluster)  [unwired: 13 in]
      n49 = Unbundle By Name(w251) -> ("Analog Data.Yokogawa.MW100"=w253:refnum<visa-resource-name>)
      n50 = call "UTILITY Aquire Semaphore.vi"("error in (no error)"=w258, "Debug"=w254, "Refnum in"=w260) -> ("error out"=w259:errorcluster, "Refnum out"=w255:T12)  [unwired: 7 in]
      n51 = call "INTELLIFAUCET Temp-Flow.vi"("Debug"=w262, "Error In"=w259, "TEMP,FLOW"="TEMP,FLOW", "VISA session"=w253) -> ("Error Out"=w257:errorcluster)  [unwired: 6 in, 1 out]
      n52 = call "UTILITY Release Semaphore.vi"("error in (no error)"=w257, "Debug"=w254, "Refnum in"=w255) -> ("error out"=w256:errorcluster)  [unwired: 8 in]
      n53 = call "INTELLIFAUCET Ready-NotReady.vi"("Refnum in"=w264, "Debug"=w265, "Error In"=w256, "READY?"=enum8{"READY", "NOT READY"}."READY", "Test Fixture Hardware"=w251) -> ("Error Out"=w272:errorcluster, "Test Fixture Hardware Output"=w273:T2)  [unwired: 5 in]
    }
  }
  "Error Out" <- w10
  "uA Output" <- w9
  "Test Fixture Hardware Output" <- w2
